vi "Object or Variant Wrapper.vi"(4 "LabVIEW Object":refnum<class>) -> (7 "Object or Variant Wrapper":refnum<class>)   [LabVIEW 2020, in "Promises.lvlib" / "Promise.lvclass"]
uses:
  Variant/Variant.lvclass
  Promise.lvclass
  Promise.lvclass/Promise.ctl
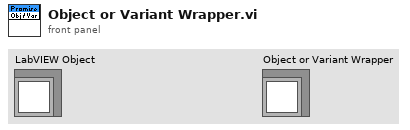
[diagram p1: front panel]
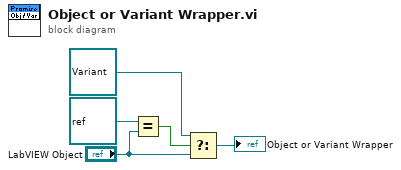
[diagram p0: block diagram]
diagram:
  n1 = Equal?(x=refnum<class> refnum, y="LabVIEW Object") -> (x = y?=w3:bool)
  n2 = Select(t=refnum<class "Variant.lvclass"> refnum ("Promises:Variant.lvclass"), s=w3, f="LabVIEW Object") -> (s? t:f=→"Object or Variant Wrapper":refnum<class>)
